vi "pix.sgl.CalcPercentiles.sgl.vi"(6 "percentiles":T1, 9 "img in":sgl[][](graph)) -> (1 "range":T2)   [LabVIEW 2020]
uses:
  _controls/cluster.range.sgl.ctl
  _controls/perc.ctl
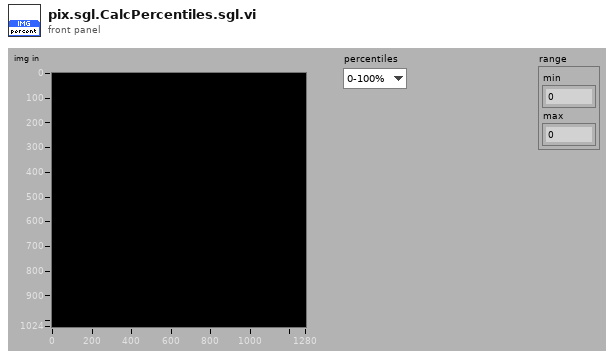
[diagram p1: front panel]
types:
  T1 = typedef "perc.ctl" = enum16{"0-100%", "1-99%", "5-95%", "10-90%", "20-80%"}
  T2 = typedef "cluster.range.sgl.ctl" = cluster{"min":sgl, "max":sgl}
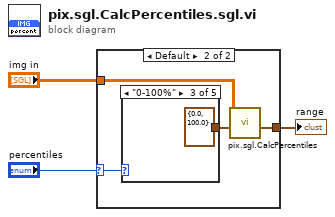
[diagram p0: block diagram]
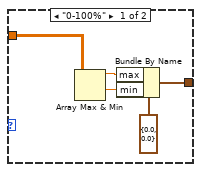
[diagram p2: hidden frame]
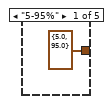
[diagram p3: hidden frame]
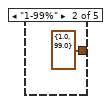
[diagram p4: hidden frame]
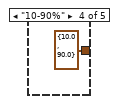
[diagram p5: hidden frame]
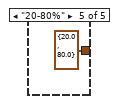
[diagram p6: hidden frame]
diagram:
  n1 = case shown="Default" "percentiles" {
    selector: "percentiles" -> [_ w11]
    tunnel: "img in" -> [w8 w10]
    tunnel: [w4 w12] -> w1
    frame "0-100%" {
      n2 = Array Max & Min(array=w8) -> (max value=w6:sgl, min value=w5:sgl)  [unwired: 2 out]
      n3 = Bundle By Name(cluster=T2 {"min"=0.0, "max"=0.0} ("range"), "max"=w6, "min"=w5) -> (w4:T2)
    }
    frame Default {
      n4 = case shown="\"0-100%\"" w11 {
        tunnel: [T2 {"min"=5.0, "max"=95.0} ("custom (1-99)") T2 {"min"=1.0, "max"=99.0} ("custom (1-99)") T2 {"min"=0.0, "max"=100.0} ("custom (1-99)") T2 {"min"=10.0, "max"=90.0} ("custom (1-99)") T2 {"min"=20.0, "max"=80.0} ("custom (1-99)")] -> w9
        frame "5-95%" {
        }
        frame "1-99%" {
        }
        frame "0-100%" {
        }
        frame "10-90%" {
        }
        frame "20-80%" {
        }
      }
      n5 = call "pix.sgl.CalcPercentiles.vi"("cutoff (%)"=w9, "pix"=w10) -> ("range"=w12:T2)  [unwired: 8 in, 1 out]
    }
  }
  "range" <- w1
